vi "VCS Get Max Profile Velocity.vi"(8 "error in (no error)":errorcluster, 11 "axis in":cluster{"keyHandle":u32, "nodeId":u16}={"keyHandle"=0, "nodeId"=1}) -> (0 "error out":errorcluster, 1 "maxProfileVelocity":u32, 3 "axis out":cluster{"keyHandle":u32, "nodeId":u16}={"keyHandle"=0, "nodeId"=1})   [LabVIEW 2010]
doc: "<B>VCS_GetMaxProfileVelocity</B> reads the maximal allowed profile velocity."
uses:
  Resources/EposCmd.dll
  Resources/EposCmd64.dll
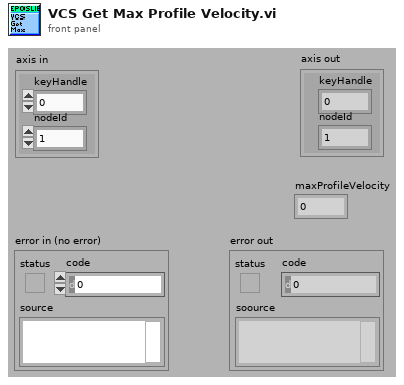
[diagram p1: front panel]
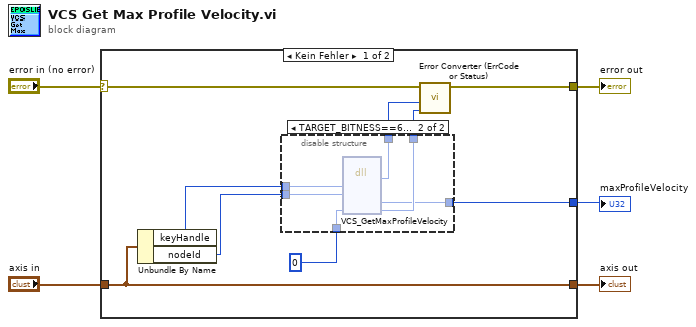
[diagram p0: block diagram]
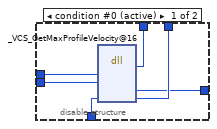
[diagram p2: hidden frame]
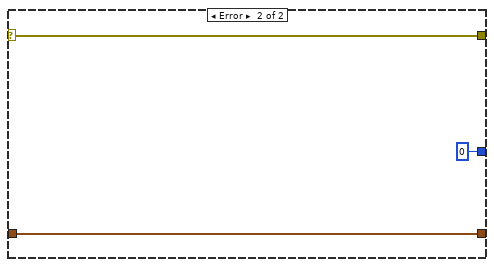
[diagram p3: hidden frame]
diagram:
  n1 = case shown="Kein Fehler" "error in (no error)" {
    selector: "error in (no error)" -> [w12 w28]
    tunnel: "axis in" -> [w14 w29]
    tunnel: [w14 w29] -> w4
    tunnel: [w13 w28] -> w3
    tunnel: [w7 u32 0 ("pMaxProfileVelocity")] -> w1
    frame No Error {
      n2 = Unbundle By Name(w14) -> ("keyHandle"=w10:u32, "nodeId"=w11:u16)
      n3 = disable-structure shown="TARGET_BITNESS==64" {
        disable-tunnel: w11 -> [w20 w26]
        disable-tunnel: w10 -> [w19 w25]
        disable-tunnel: [w18 w24] -> w9
        disable-tunnel: [w17 w23] -> w8
        disable-tunnel: [w16 w22] -> w7
        disable-tunnel: u32 0 ("pErrorCode") -> [w15 w21]
        frame condition #0 (active) {
          n4 = dll-call lib="C:/Sources/LabView/maxon EPOS/Resources/EposCmd.*" fn="_VCS_GetMaxProfileVelocity@16"("KeyHandle"=w19, "NodeId"=w20, "pErrorCode"=w15) -> (w18:i32, "pMaxProfileVelocity"=w16:u32, "pErrorCode"=w17:u32)  [unwired: 6 in, 2 out]
        }
        frame condition #1 {
          n5 = dll-call lib="C:/setup/Resources/EposCmd64.*" fn="VCS_GetMaxProfileVelocity" ("EposCmd.dll:_VCS_GetMaxProfileVelocity@16")("KeyHandle"=w25, "NodeId"=w26, "pErrorCode"=w21) -> ("Rückgabetyp"=w24:i32, "pMaxProfileVelocity"=w22:u32, "pErrorCode"=w23:u32)  [unwired: 6 in, 2 out]
        }
      }
      n6 = call "Error Converter (ErrCode or Status).vi"("error code"=w8, "return type"=w9, "error in (no error)"=w12) -> ("error out"=w13:errorcluster)  [unwired: 7 in]
    }
    frame Error {
    }
  }
  "maxProfileVelocity" <- w1
  "error out" <- w3
  "axis out" <- w4
